vi "3-9.vi"() -> ()   [LabVIEW 2014]
panel:
  in  "Max Wind Speed":dbl
  in  "Current Wind Speed":dbl
  out "Warning Text":string
  out "Warning?":bool
  in  "Min Temp":dbl
  in  "Max Temp":dbl
  in  "Current Temp":dbl
  # "You must create a portion of a larger project. The lead developer gives you the inputs of the VI, the\nalgorithm, and the expected outputs. Create and document a VI based on the given design."
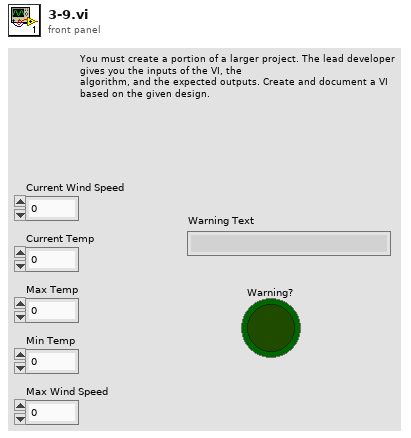
[diagram p1: front panel]
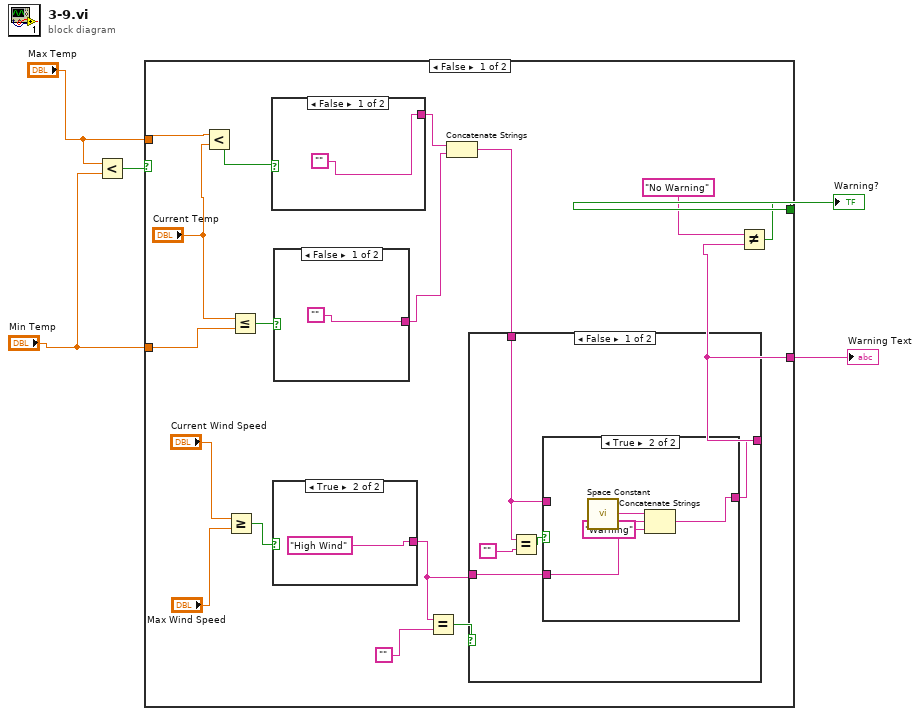
[diagram p0: block diagram]
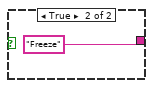
[diagram p2: hidden frame]
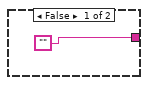
[diagram p3: hidden frame]
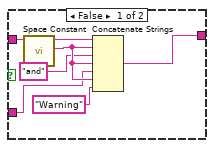
[diagram p4: hidden frame]
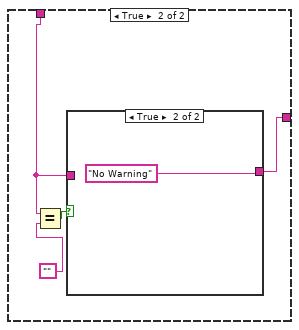
[diagram p5: hidden frame]
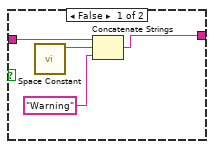
[diagram p6: hidden frame]
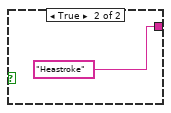
[diagram p7: hidden frame]
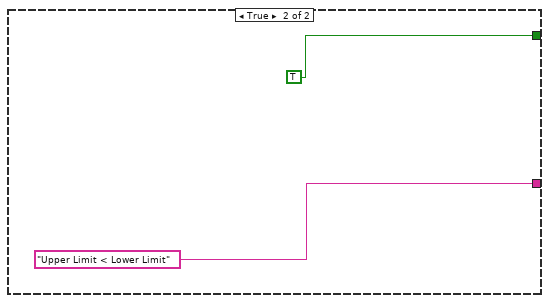
[diagram p8: hidden frame]
diagram:
  n1 = Less?(x="Max Temp", y="Min Temp") -> (x < y?=w4:bool)
  n2 = case shown="False" w4 {
    tunnel: [w22 TRUE] -> w5
    tunnel: "Min Temp" -> [w21 _]
    tunnel: "Max Temp" -> [w19 _]
    tunnel: [w7 "Upper Limit < Lower Limit"] -> w3
    frame False {
      n3 = Less?(x=w19, y="Current Temp") -> (x < y?=w20:bool)
      n4 = Greater Or Equal?(x="Current Wind Speed", y="Max Wind Speed") -> (x >= y?=w14:bool)
      n5 = Less Or Equal?(x="Current Temp", y=w21) -> (x <= y?=w10:bool)
      n6 = case shown="False" w20 {
        tunnel: ["" "Heastroke"] -> w17
        frame False {
        }
        frame True {
        }
      }
      n7 = case shown="True" w14 {
        tunnel: ["" "High Wind"] -> w11
        frame False {
        }
        frame True {
        }
      }
      n8 = case shown="False" w10 {
        tunnel: ["" "Freeze"] -> w9
        frame False {
        }
        frame True {
        }
      }
      n9 = Equal?(x=w11, y="") -> (x = y?=w13:bool)
      n10 = Concatenate Strings(w17, w9) -> (w6:string)
      n11 = case shown="False" w13 {
        tunnel: [w27 w43] -> w7
        tunnel: w11 -> [w29 _]
        tunnel: w6 -> [w28 w42]
        frame False {
          n12 = Equal?(x=w28, y="") -> (x = y?=w31:bool)
          n13 = case shown="True" w31 {
            tunnel: [w37 w38] -> w27
            tunnel: w29 -> [w32 w40]
            tunnel: w28 -> [w36 _]
            frame False {
              n14 = call <vilib>:"Space Constant.vi"() -> ("String"=w35:string)
              n15 = Concatenate Strings(w36, w35, "and" ("string"), w35, w32, w35, "Warning") -> (w37:string)
            }
            frame True {
              n16 = call <vilib>:"Space Constant.vi"() -> ("String"=w41:string)
              n17 = Concatenate Strings(w40, w41, "Warning" ("string")) -> (w38:string)
            }
          }
        }
        frame True {
          n18 = Equal?(x=w42, y="") -> (x = y?=w45:bool)
          n19 = case shown="True" w45 {
            tunnel: [w47 "No Warning"] -> w43
            tunnel: w42 -> [w46 _]
            frame False {
              n20 = call <vilib>:"Space Constant.vi"() -> ("String"=w49:string)
              n21 = Concatenate Strings(w46, w49, "Warning") -> (w47:string)
            }
            frame True {
            }
          }
        }
      }
      n22 = Not Equal?(x="No Warning", y=w7) -> (x != y?=w22:bool)
    }
    frame True {
    }
  }
  "Warning?" <- w5
  "Warning Text" <- w3
